vi "Transfer Packets From Host.vi"(1 "reset":bool, 2 "common resources":T13={"sync pulse resources"={"sync pulse destination terminal"="", "sync100"="", "sync pulse source terminal"="", "imported sync pulse register"="", "generate sync pulse handshake"="", "enable sync pulse register"="", "sync pulse clock"=""}, "serial channel resources"={"sc 0"={"completed frames register"=""}, "sc 1"={"completed frames register"=""}, "sc 2"={"completed frames register"=""}, "sc 3"={"completed frames register"=""}, "sc 4"={"completed frames register"=""}, "sc 5"={"completed frames register"=""}, "sc 6"={"completed frames register"=""}, "sc 7"={"completed frames register"=""}}, "dram manager 0"={"DRAM class"=refnum, "process clock"="", "registers"={"configuration"={"write time slice"="", "request time slice"="", "DRAM arbiter config"="", "partition config"=""}, "reset"={"handshake"={"start.go"="", "start.go rcvd"="", "done.go"="", "done.go rcvd"=""}, "process"={"in"="", "out"=""}, "write"={"in"="", "out 0"="", "out 1"="", "out 2"="", "out 3"=""}, "read"={"in"="", "out 0"="", "out 1"="", "out 2"="", "out 3"=""}}, "status"={"partition full"=""}}, "FIFOs"={"write data"={"FIFO 0"="", "FIFO 1"="", "FIFO 2"="", "FIFO 3"=""}, "request metadata"={"FIFO"=""}, "read data VOQ"={"FIFO 0"="", "FIFO 1"="", "FIFO 2"="", "FIFO 3"=""}, "read data"={"FIFO 0"="", "FIFO 1"="", "FIFO 2"="", "FIFO 3"=""}}, "num active streams"=0.0, "max open read requests"=256}, "dram manager 1"={"DRAM class"=refnum, "process clock"="", "registers"={"configuration"={"write time slice"="", "request time slice"="", "DRAM arbiter config"="", "partition config"=""}, "reset"={"handshake"={"start.go"="", "start.go rcvd"="", "done.go"="", "done.go rcvd"=""}, "process"={"in"="", "out"=""}, "write"={"in"="", "out 0"="", "out 1"="", "out 2"="", "out 3"=""}, "read"={"in"="", "out 0"="", "out 1"="", "out 2"="", "out 3"=""}}, "status"={"partition full"=""}}, "FIFOs"={"write data"={"FIFO 0"="", "FIFO 1"="", "FIFO 2"="", "FIFO 3"=""}, "request metadata"={"FIFO"=""}, "read data VOQ"={"FIFO 0"="", "FIFO 1"="", "FIFO 2"="", "FIFO 3"=""}, "read data"={"FIFO 0"="", "FIFO 1"="", "FIFO 2"="", "FIFO 3"=""}}, "num active streams"=0.0, "max open read requests"=256}}, 11 "dram partition configs":T12[](array[typedef])=[{"first address"=0, "last address"=0}, {"first address"=0, "last address"=0}, {"first address"=0, "last address"=0}, {"first address"=0, "last address"=0}, {"first address"=0, "last address"=0}, {"first address"=0, "last address"=0}, {"first address"=0, "last address"=0}, {"first address"=0, "last address"=0}], 12 "ready for output":bool[](array[boolean])=[TRUE, TRUE, TRUE, TRUE, TRUE, TRUE, TRUE, TRUE], 13 "channel configs":T24[](array[typedef])) -> (4 "tagged llp packets cluster":T1, 6 "end of data":bool[](array[boolean]), 8 "dram status":T11[](array[typedef]), 10 "output valid":bool[](array[boolean]))   [LabVIEW 2020, in "GettingStarted_Gen_148X_FPGA.lvlib"]
uses:
  GettingStarted_Gen_148X_FPGA.lvlib
  Types/Serial Output Channel Datapath Configuration.ctl
  Common/Types/Common Resources.ctl
  <instrlib>/_niInstr/Memory/v1/FPGA/DRAM/niInstr Memory DRAM v1 FPGA.lvclass
  <instrlib>/FlexRIO/CSI-2/v2/FPGA/Types/Sync Pulse Resources.ctl
  Common/Types/Serial Channel Resources.ctl
  Common/Types/Single Serial Channel Resources.ctl
  <instrlib>/FlexRIO/CSI-2/v2/FPGA/DRAM Manager/Private/DRAM Manager.ctl
  <instrlib>/FlexRIO/CSI-2/v2/FPGA/DRAM Manager/Private/Common/DRAM Manager Registers.ctl
  <instrlib>/FlexRIO/CSI-2/v2/FPGA/DRAM Manager/Private/Common/Handshake Registers.ctl
  <instrlib>/FlexRIO/CSI-2/v2/FPGA/DRAM Manager/Private/Common/DRAM Manager FIFOs.ctl
  <instrlib>/FlexRIO/CSI-2/v2/FPGA/DRAM Manager/Private/Common/Write Data FIFO Ref.ctl
  <instrlib>/FlexRIO/CSI-2/v2/FPGA/DRAM Manager/Private/Common/Read Request Metadata FIFO Ref.ctl
  <instrlib>/FlexRIO/CSI-2/v2/FPGA/DRAM Manager/Private/Common/Read Data FIFO Ref.ctl
  <instrlib>/FlexRIO/CSI-2/v2/FPGA/DRAM Manager/Public/Partition Range.ctl
  Common/Types/DRAM Status.ctl
  Common/Types/Tagged LLP Packets Cluster.ctl
  <instrlib>/FlexRIO/CSI-2/v2/FPGA/Types/Tagged LLP Packet.ctl
  <instrlib>/FlexRIO/CSI-2/v2/FPGA/Types/FPGA LLP Packet Tag.ctl
  <instrlib>/FlexRIO/CSI-2/v2/FPGA/Types/FPGA LLP Packet Timestamp.ctl
  <instrlib>/FlexRIO/CSI-2/v2/FPGA/Types/Timestamp ID.ctl
  <instrlib>/FlexRIO/CSI-2/v2/FPGA/Types/FPGA LLP Packet Size.ctl
  <instrlib>/FlexRIO/CSI-2/v2/FPGA/Types/LLP Packet.ctl
  <instrlib>/FlexRIO/CSI-2/v2/FPGA/Types/LLP Packet Header.ctl
  <instrlib>/FlexRIO/CSI-2/v2/FPGA/Types/LLP Packet Payload.ctl
  <instrlib>/FlexRIO/CSI-2/v2/FPGA/Types/LLP Packet Footer.ctl
  <instrlib>/_niInstr/Basic Elements/v1/FPGA/niInstr Basic Elements v1 FPGA.lvlib
  <instrlib>/FlexRIO/CSI-2/v2/FPGA/NI CSI-2 API FPGA v2.lvlib
  Common/GettingStarted_Common_148X_FPGA.lvlib
  <instrlib>/FlexRIO/CSI-2/v2/FPGA/DRAM Manager/DRAM Manager v2.lvlib
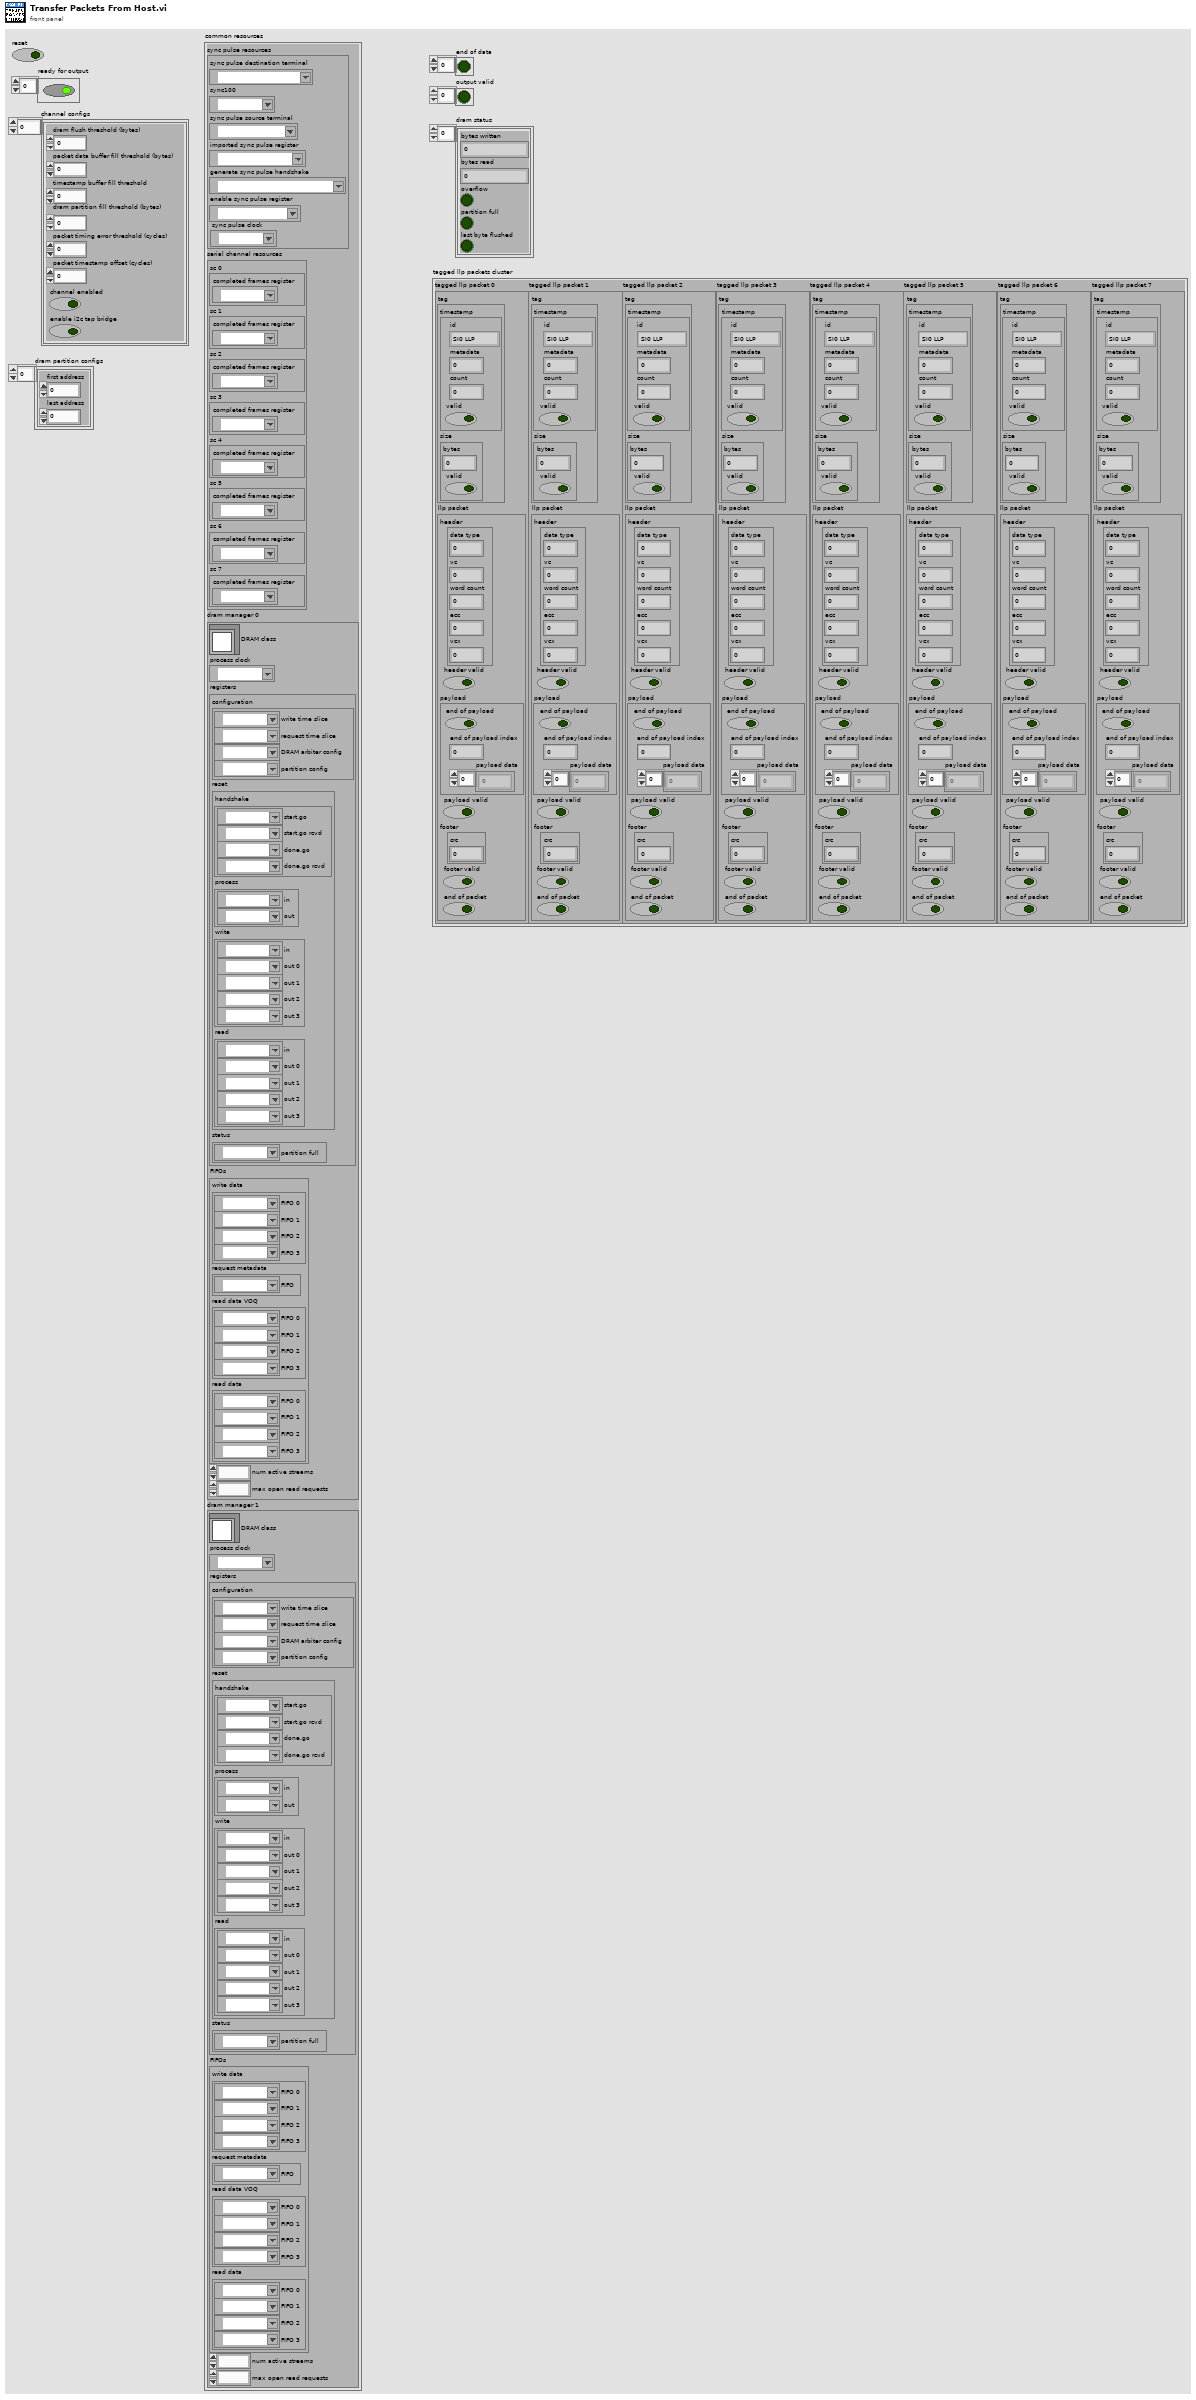
[diagram p1: front panel]
types:
  T1 = typedef "GettingStarted_Common_148X_FPGA.lvlib/Tagged LLP Packets Cluster.ctl" = cluster{"tagged llp packet 0":T2, "tagged llp packet 1":T2, "tagged llp packet 2":T2, "tagged llp packet 3":T2, "tagged llp packet 4":T2, "tagged llp packet 5":T2, "tagged llp packet 6":T2, "tagged llp packet 7":T2}
  T2 = typedef "NI CSI-2 API FPGA v2.lvlib/Tagged LLP Packet.ctl" = cluster{"tag":T3, "llp packet":T7}
  T3 = typedef "NI CSI-2 API FPGA v2.lvlib/FPGA LLP Packet Tag.ctl" = cluster{"timestamp":T4, "size":T6}
  T4 = typedef "NI CSI-2 API FPGA v2.lvlib/FPGA LLP Packet Timestamp.ctl" = cluster{"valid":bool, "count":fxp<+,50,50>, "id":T5, "metadata":u8}
  T5 = typedef "NI CSI-2 API FPGA v2.lvlib/Timestamp ID.ctl" = enum8{"SI0 LLP", "SI1 LLP", "SI2 LLP", "SI3 LLP", "SI4 LLP", "SI5 LLP", "SI6 LLP", "SI7 LLP", "SO0 LLP", "SO1 LLP", "SO2 LLP", "SO3 LLP", "SO4 LLP", "SO5 LLP", "SO6 LLP", "SO7 LLP", "Ser0 GPIO Bank", "Ser1 GPIO Bank", "Ser2 GPIO Bank", "Ser3 GPIO Bank", "Ser4 GPIO Bank", "Ser5 GPIO Bank", "Ser6 GPIO Bank", "Ser7 GPIO Bank", "Des0 GPIO Bank", "Des1 GPIO Bank", "Des2 GPIO Bank", "Des3 GPIO Bank", "Des4 GPIO Bank", "Des5 GPIO Bank", "Des6 GPIO Bank", "Des7 GPIO Bank", "User0", "User1", "User2", "User3", "User4", "User5", "User6", "User7", "User8", "User9", "User10", "User11", "User12", "User13", "User14", "User15", "User16", "User17", "User18", "User19", "User20", "User21", "User22", "User23", "User24", "User25", "User26", "User27", "User28", "User29", "User30", "User31"}
  T6 = typedef "NI CSI-2 API FPGA v2.lvlib/FPGA LLP Packet Size.ctl" = cluster{"bytes":fxp<+,17,17>, "valid":bool}
  T7 = typedef "NI CSI-2 API FPGA v2.lvlib/LLP Packet.ctl" = cluster{"header":T8, "header valid":bool, "payload":T9, "payload valid":bool, "footer":T10, "footer valid":bool, "end of packet":bool}
  T8 = typedef "NI CSI-2 API FPGA v2.lvlib/LLP Packet Header.ctl" = cluster{"word count":u16, "ecc":fxp<+,6,6>, "vcx":fxp<+,2,2>, "data type":fxp<+,6,6>, "vc":fxp<+,2,2>}
  T9 = typedef "NI CSI-2 API FPGA v2.lvlib/LLP Packet Payload.ctl" = cluster{"end of payload":bool, "end of payload index":fxp<+,3,3>, "payload data":u8[]}
  T10 = typedef "NI CSI-2 API FPGA v2.lvlib/LLP Packet Footer.ctl" = cluster{"crc":u16}
  T11 = typedef "GettingStarted_Common_148X_FPGA.lvlib/DRAM Status.ctl" = cluster{"bytes written":u64, "bytes read":u64, "overflow":bool, "partition full":bool, "last byte flushed":bool}
  T12 = typedef "DRAM Manager v2.lvlib/Partition Range.ctl" = cluster{"first address":u32, "last address":u32}
  T13 = typedef "GettingStarted_Common_148X_FPGA.lvlib/Common Resources.ctl" = cluster{"sync pulse resources":T14, "serial channel resources":T15, "dram manager 0":T17, "dram manager 1":T17}
  T14 = typedef "NI CSI-2 API FPGA v2.lvlib/Sync Pulse Resources.ctl" = cluster{"sync pulse destination terminal":refnum<k21>, "sync100":refnum<k21>, "sync pulse source terminal":refnum<k21>, "imported sync pulse register":refnum<k21>, "generate sync pulse handshake":refnum<k21>, "enable sync pulse register":refnum<k21>, "sync pulse clock":refnum<k21>}
  T15 = typedef "GettingStarted_Common_148X_FPGA.lvlib/Serial Channel Resources.ctl" = cluster{"sc 0":T16, "sc 1":T16, "sc 2":T16, "sc 3":T16, "sc 4":T16, "sc 5":T16, "sc 6":T16, "sc 7":T16}
  T16 = typedef "GettingStarted_Common_148X_FPGA.lvlib/Single Serial Channel Resources.ctl" = cluster{"completed frames register":refnum<k21>}
  T17 = typedef "DRAM Manager v2.lvlib/DRAM Manager.ctl" = cluster{"DRAM class":refnum<class "niInstr Memory DRAM v1 FPGA.lvclass">, "process clock":refnum<k21>, "registers":T18, "FIFOs":T20, "num active streams":fxp<+,3,3>, "max open read requests":u16}
  T18 = typedef "DRAM Manager v2.lvlib/DRAM Manager Registers.ctl" = cluster{"configuration":cluster{"write time slice":refnum<k21>, "request time slice":refnum<k21>, "DRAM arbiter config":refnum<k21>, "partition config":refnum<k21>}, "reset":cluster{"handshake":T19, "process":cluster{"in":refnum<k21>, "out":refnum<k21>}, "write":cluster{"in":refnum<k21>, "out 0":refnum<k21>, "out 1":refnum<k21>, "out 2":refnum<k21>, "out 3":refnum<k21>}, "read":cluster{"in":refnum<k21>, "out 0":refnum<k21>, "out 1":refnum<k21>, "out 2":refnum<k21>, "out 3":refnum<k21>}}, "status":cluster{"partition full":refnum<k21>}}
  T19 = typedef "DRAM Manager v2.lvlib/Handshake Registers.ctl" = cluster{"start.go":refnum<k21>, "start.go rcvd":refnum<k21>, "done.go":refnum<k21>, "done.go rcvd":refnum<k21>}
  T20 = typedef "DRAM Manager v2.lvlib/DRAM Manager FIFOs.ctl" = cluster{"write data":cluster{"FIFO 0":T21, "FIFO 1":T21, "FIFO 2":T21, "FIFO 3":T21}, "request metadata":cluster{"FIFO":T22}, "read data VOQ":cluster{"FIFO 0":T23, "FIFO 1":T23, "FIFO 2":T23, "FIFO 3":T23}, "read data":cluster{"FIFO 0":T23, "FIFO 1":T23, "FIFO 2":T23, "FIFO 3":T23}}
  T21 = typedef "DRAM Manager v2.lvlib/Write Data FIFO Ref.ctl" = refnum<k21>
  T22 = typedef "DRAM Manager v2.lvlib/Read Request Metadata FIFO Ref.ctl" = refnum<k21>
  T23 = typedef "DRAM Manager v2.lvlib/Read Data FIFO Ref.ctl" = refnum<k21>
  T24 = typedef "GettingStarted_Gen_148X_FPGA.lvlib/Serial Output Channel Datapath Configuration.ctl" = cluster{"dram flush threshold (bytes)":u64, "packet data buffer fill threshold (bytes)":u64, "timestamp buffer fill threshold":u32, "packet timing error threshold (cycles)":u64, "channel enabled":bool, "dram partition fill threshold (bytes)":u64, "enable i2c tap bridge":bool, "packet timestamp offset (cycles)":i64}
  T25 = typedef "GettingStarted_Gen_148X_FPGA.lvlib/8 Out DRAM Resources.ctl" = cluster{"so 0 resources":T26, "so 1 resources":T26, "so 2 resources":T26, "so 3 resources":T26, "so 4 resources":T26, "so 5 resources":T26, "so 6 resources":T26, "so 7 resources":T26}
  T26 = typedef "GettingStarted_Gen_148X_FPGA.lvlib/Serial Output DRAM Resources.ctl" = cluster{"dram manager":T17, "llp packets dma fifo":refnum<k21>, "dram stream id":fxp<+,2,2>}
  T27 = cluster{"end of data":bool, "dram status":T11, "output valid":bool}
  T28 = cluster{"end of data":bool, "dram status":T11, "output valid":bool}[]
  T29 = typedef "GettingStarted_Gen_148X_FPGA.lvlib/4 In 4 Out DRAM Resources.ctl" = cluster{"so 0 resources":T26, "so 1 resources":T26, "so 2 resources":T26, "so 3 resources":T26}
  T30 = typedef "GettingStarted_Gen_148X_FPGA.lvlib/2 In 2 Out DRAM Resources.ctl" = cluster{"so 0 resources":T26, "so 1 resources":T26}
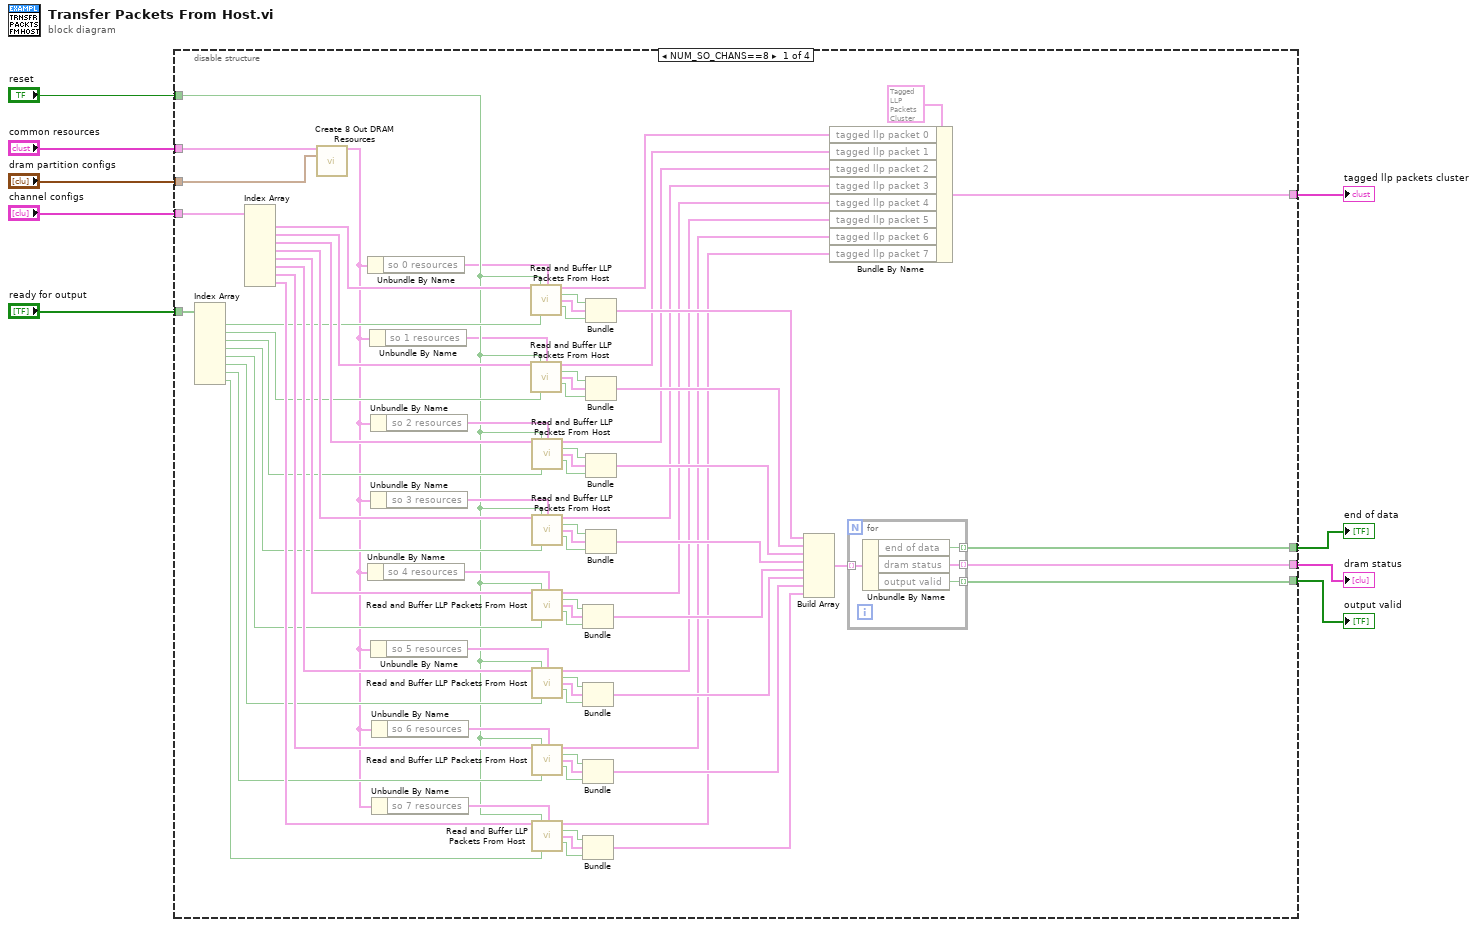
[diagram p0: block diagram]
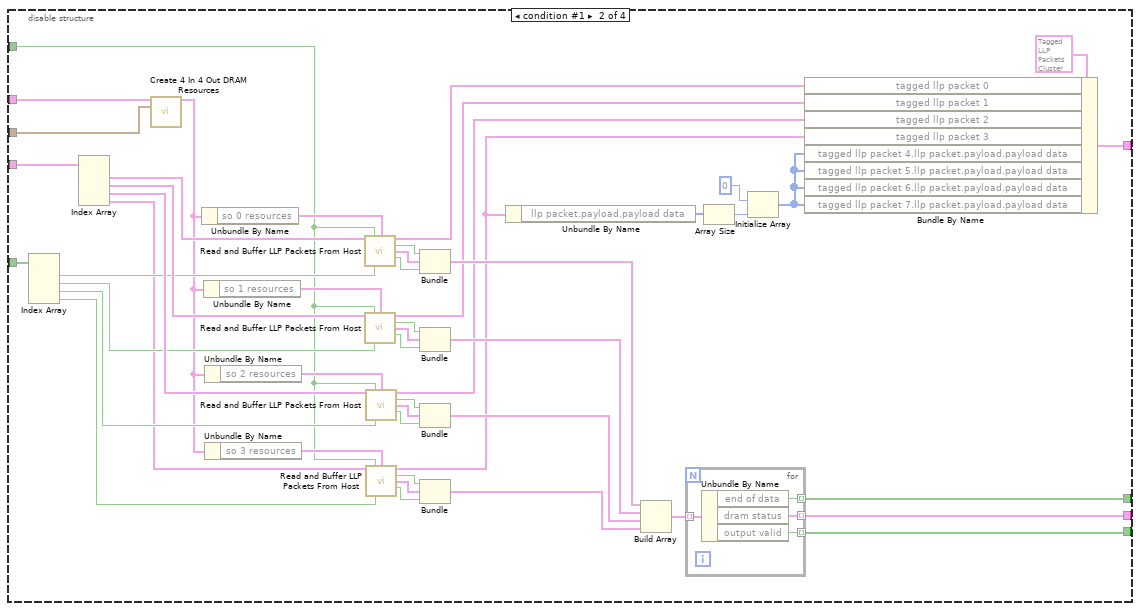
[diagram p2: hidden frame]
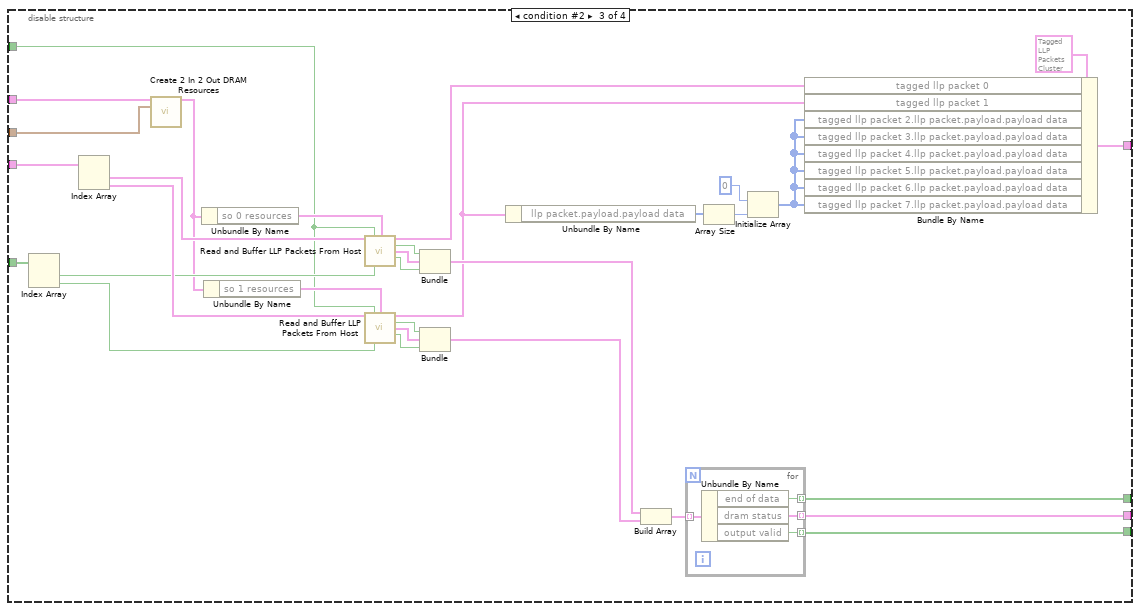
[diagram p3: hidden frame]
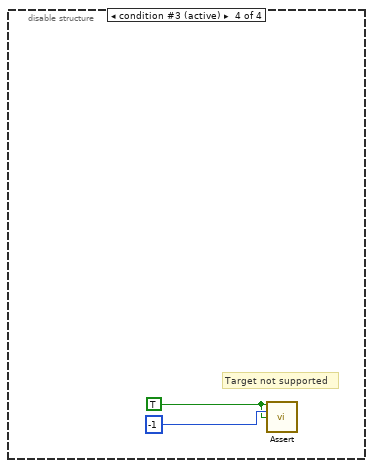
[diagram p4: hidden frame]
diagram:
  n1 = disable-structure shown="NUM_SO_CHANS==8" {
    disable-tunnel: "channel configs" -> [w85 w137 w173 _]
    disable-tunnel: "common resources" -> [w60 w125 w164 _]
    disable-tunnel: "dram partition configs" -> [w61 w126 w165 _]
    disable-tunnel: "ready for output" -> [w84 w136 w172 _]
    disable-tunnel: [w25 w110 w153 _] -> w6
    disable-tunnel: "reset" -> [w24 w102 w152 _]
    disable-tunnel: [w21 w100 w150 _] -> w3
    disable-tunnel: [w20 w101 w151 _] -> w2
    disable-tunnel: [w10 w98 w148 _] -> w1
    frame condition #0 {
      n2 = Index Array(array=w84) -> (element #1=w69:bool, element #2=w68:bool, element #3=w62:bool, element #4=w63:bool, element #5=w64:bool, element #6=w65:bool, element #7=w66:bool, element #8=w67:bool)  [unwired: 8 in]
      n3 = Index Array(array=w85) -> (element #1=w83:T24, element #2=w82:T24, element #3=w80:T24, element #4=w81:T24, element #5=w70:T24, element #6=w71:T24, element #7=w72:T24, element #8=w73:T24)  [unwired: 8 in]
      n4 = call "Create 8 Out DRAM Resources.vi"("common resources"=w60, "dram partition configs"=w61) -> ("channel dram resources"=w59:T25)  [unwired: 13 in]
      n5 = Unbundle By Name(w59) -> ("so 0 resources"=w23:T26)
      n6 = Unbundle By Name(w59) -> ("so 4 resources"=w77:T26)
      n7 = Unbundle By Name(w59) -> ("so 1 resources"=w22:T26)
      n8 = Unbundle By Name(w59) -> ("so 2 resources"=w79:T26)
      n9 = Unbundle By Name(w59) -> ("so 3 resources"=w78:T26)
      n10 = Unbundle By Name(w59) -> ("so 5 resources"=w76:T26)
      n11 = Unbundle By Name(w59) -> ("so 6 resources"=w75:T26)
      n12 = Unbundle By Name(w59) -> ("so 7 resources"=w74:T26)
      n13 = call "Read and Buffer LLP Packets From Host.vi"("channel configuration"=w83, "reset"=w24, "resources"=w23, "ready for output"=w69) -> ("tagged llp packet"=w11:T2, "end of data"=w58:bool, "dram status"=w57:T11, "output valid"=w56:bool)  [unwired: 8 in]
      n14 = call "Read and Buffer LLP Packets From Host.vi"("channel configuration"=w82, "reset"=w24, "resources"=w22, "ready for output"=w68) -> ("tagged llp packet"=w12:T2, "end of data"=w53:bool, "dram status"=w54:T11, "output valid"=w55:bool)  [unwired: 8 in]
      n15 = call "Read and Buffer LLP Packets From Host.vi"("channel configuration"=w80, "reset"=w24, "resources"=w79, "ready for output"=w62) -> ("tagged llp packet"=w13:T2, "end of data"=w52:bool, "dram status"=w51:T11, "output valid"=w50:bool)  [unwired: 8 in]
      n16 = call "Read and Buffer LLP Packets From Host.vi"("channel configuration"=w81, "reset"=w24, "resources"=w78, "ready for output"=w63) -> ("tagged llp packet"=w14:T2, "end of data"=w49:bool, "dram status"=w48:T11, "output valid"=w47:bool)  [unwired: 8 in]
      n17 = call "Read and Buffer LLP Packets From Host.vi"("channel configuration"=w70, "reset"=w24, "resources"=w77, "ready for output"=w64) -> ("tagged llp packet"=w15:T2, "end of data"=w46:bool, "dram status"=w45:T11, "output valid"=w44:bool)  [unwired: 8 in]
      n18 = call "Read and Buffer LLP Packets From Host.vi"("channel configuration"=w71, "reset"=w24, "resources"=w76, "ready for output"=w65) -> ("tagged llp packet"=w16:T2, "end of data"=w43:bool, "dram status"=w42:T11, "output valid"=w41:bool)  [unwired: 8 in]
      n19 = call "Read and Buffer LLP Packets From Host.vi"("channel configuration"=w72, "reset"=w24, "resources"=w75, "ready for output"=w66) -> ("tagged llp packet"=w17:T2, "end of data"=w40:bool, "dram status"=w39:T11, "output valid"=w38:bool)  [unwired: 8 in]
      n20 = call "Read and Buffer LLP Packets From Host.vi"("channel configuration"=w73, "reset"=w24, "resources"=w74, "ready for output"=w67) -> ("tagged llp packet"=w18:T2, "end of data"=w37:bool, "dram status"=w36:T11, "output valid"=w35:bool)  [unwired: 8 in]
      n21 = Bundle("end of data"=w46, "dram status"=w45, "output valid"=w44) -> (w30:T27)  [unwired: 1 in]
      n22 = Bundle("end of data"=w43, "dram status"=w42, "output valid"=w41) -> (w29:T27)  [unwired: 1 in]
      n23 = Bundle("end of data"=w40, "dram status"=w39, "output valid"=w38) -> (w28:T27)  [unwired: 1 in]
      n24 = Bundle("end of data"=w37, "dram status"=w36, "output valid"=w35) -> (w27:T27)  [unwired: 1 in]
      n25 = Bundle("end of data"=w58, "dram status"=w57, "output valid"=w56) -> (w34:T27)  [unwired: 1 in]
      n26 = Bundle("end of data"=w53, "dram status"=w54, "output valid"=w55) -> (w33:T27)  [unwired: 1 in]
      n27 = Bundle("end of data"=w52, "dram status"=w51, "output valid"=w50) -> (w32:T27)  [unwired: 1 in]
      n28 = Bundle("end of data"=w49, "dram status"=w48, "output valid"=w47) -> (w31:T27)  [unwired: 1 in]
      n29 = Build Array(w34, w33, w32, w31, w30, w29, w28, w27) -> (w26:T28)
      n30 = Bundle By Name(cluster=T1 {"tagged llp packet 0"={"tag"={"timestamp"={"valid"=FALSE, "count"=0.0, "id"=enum."SI0 LLP", "metadata"=0}, "size"={"bytes"=0.0, "valid"=FALSE}}, "llp packet"={"header"={"word count"=0, "ecc"=0.0, "vcx"=0.0, "data type"=0.0, "vc"=0.0}, "header valid"=FALSE, "payload"={"end of payload"=FALSE, "end of payload index"=0.0, "payload data"=[0, 0, 0, 0]}, "payload valid"=FALSE, "footer"={"crc"=0}, "footer valid"=FALSE, "end of packet"=FALSE}}, "tagged llp packet 1"={"tag"={"timestamp"={"valid"=FALSE, "count"=0.0, "id"=enum."SI0 LLP", "metadata"=0}, "size"={"bytes"=0.0, "valid"=FALSE}}, "llp packet"={"header"={"word count"=0, "ecc"=0.0, "vcx"=0.0, "data type"=0.0, "vc"=0.0}, "header valid"=FALSE, "payload"={"end of payload"=FALSE, "end of payload index"=0.0, "payload data"=[0, 0, 0, 0]}, "payload valid"=FALSE, "footer"={"crc"=0}, "footer valid"=FALSE, "end of packet"=FALSE}}, "tagged llp packet 2"={"tag"={"timestamp"={"valid"=FALSE, "count"=0.0, "id"=enum."SI0 LLP", "metadata"=0}, "size"={"bytes"=0.0, "valid"=FALSE}}, "llp packet"={"header"={"word count"=0, "ecc"=0.0, "vcx"=0.0, "data type"=0.0, "vc"=0.0}, "header valid"=FALSE, "payload"={"end of payload"=FALSE, "end of payload index"=0.0, "payload data"=[0, 0, 0, 0]}, "payload valid"=FALSE, "footer"={"crc"=0}, "footer valid"=FALSE, "end of packet"=FALSE}}, "tagged llp packet 3"={"tag"={"timestamp"={"valid"=FALSE, "count"=0.0, "id"=enum."SI0 LLP", "metadata"=0}, "size"={"bytes"=0.0, "valid"=FALSE}}, "llp packet"={"header"={"word count"=0, "ecc"=0.0, "vcx"=0.0, "data type"=0.0, "vc"=0.0}, "header valid"=FALSE, "payload"={"end of payload"=FALSE, "end of payload index"=0.0, "payload data"=[0, 0, 0, 0]}, "payload valid"=FALSE, "footer"={"crc"=0}, "footer valid"=FALSE, "end of packet"=FALSE}}, "tagged llp packet 4"={"tag"={"timestamp"={"valid"=FALSE, "count"=0.0, "id"=enum."SI0 LLP", "metadata"=0}, "size"={"bytes"=0.0, "valid"=FALSE}}, "llp packet"={"header"={"word count"=0, "ecc"=0.0, "vcx"=0.0, "data type"=0.0, "vc"=0.0}, "header valid"=FALSE, "payload"={"end of payload"=FALSE, "end of payload index"=0.0, "payload data"=[0, 0, 0, 0]}, "payload valid"=FALSE, "footer"={"crc"=0}, "footer valid"=FALSE, "end of packet"=FALSE}}, "tagged llp packet 5"={"tag"={"timestamp"={"valid"=FALSE, "count"=0.0, "id"=enum."SI0 LLP", "metadata"=0}, "size"={"bytes"=0.0, "valid"=FALSE}}, "llp packet"={"header"={"word count"=0, "ecc"=0.0, "vcx"=0.0, "data type"=0.0, "vc"=0.0}, "header valid"=FALSE, "payload"={"end of payload"=FALSE, "end of payload index"=0.0, "payload data"=[0, 0, 0, 0]}, "payload valid"=FALSE, "footer"={"crc"=0}, "footer valid"=FALSE, "end of packet"=FALSE}}, "tagged llp packet 6"={"tag"={"timestamp"={"valid"=FALSE, "count"=0.0, "id"=enum."SI0 LLP", "metadata"=0}, "size"={"bytes"=0.0, "valid"=FALSE}}, "llp packet"={"header"={"word count"=0, "ecc"=0.0, "vcx"=0.0, "data type"=0.0, "vc"=0.0}, "header valid"=FALSE, "payload"={"end of payload"=FALSE, "end of payload index"=0.0, "payload data"=[0, 0, 0, 0]}, "payload valid"=FALSE, "footer"={"crc"=0}, "footer valid"=FALSE, "end of packet"=FALSE}}, "tagged llp packet 7"={"tag"={"timestamp"={"valid"=FALSE, "count"=0.0, "id"=enum."SI0 LLP", "metadata"=0}, "size"={"bytes"=0.0, "valid"=FALSE}}, "llp packet"={"header"={"word count"=0, "ecc"=0.0, "vcx"=0.0, "data type"=0.0, "vc"=0.0}, "header valid"=FALSE, "payload"={"end of payload"=FALSE, "end of payload index"=0.0, "payload data"=[0, 0, 0, 0]}, "payload valid"=FALSE, "footer"={"crc"=0}, "footer valid"=FALSE, "end of packet"=FALSE}}} ("tagged llp packets cluster"), "tagged llp packet 0"=w11, "tagged llp packet 1"=w12, "tagged llp packet 2"=w13, "tagged llp packet 3"=w14, "tagged llp packet 4"=w15, "tagged llp packet 5"=w16, "tagged llp packet 6"=w17, "tagged llp packet 7"=w18) -> (w10:T1)
      n31 = for {
        tunnel: w26 -> [w89] mode=indexing
        tunnel: [w88] -> w20 mode=indexing
        tunnel: [w87] -> w25 mode=indexing
        tunnel: [w86] -> w21 mode=indexing
        n32 = Unbundle By Name(w89) -> ("end of data"=w88:bool, "dram status"=w87:T11, "output valid"=w86:bool)
      }
    }
    frame condition #1 {
      n33 = Index Array(array=w136) -> (element #1=w129:bool, element #2=w128:bool, element #3=w127:bool, element #4=w103:bool)  [unwired: 4 in]
      n34 = Index Array(array=w137) -> (element #1=w134:T24, element #2=w132:T24, element #3=w131:T24, element #4=w106:T24)  [unwired: 4 in]
      n35 = call "Create 4 In 4 Out DRAM Resources.vi"("common resources"=w125, "dram partition configs"=w126) -> ("channel dram resources"=w124:T29)  [unwired: 13 in]
      n36 = Unbundle By Name(w124) -> ("so 0 resources"=w135:T26)
      n37 = Unbundle By Name(w124) -> ("so 1 resources"=w133:T26)
      n38 = Unbundle By Name(w124) -> ("so 2 resources"=w130:T26)
      n39 = Unbundle By Name(w124) -> ("so 3 resources"=w104:T26)
      n40 = call "Read and Buffer LLP Packets From Host.vi"("channel configuration"=w134, "reset"=w102, "resources"=w135, "ready for output"=w129) -> ("tagged llp packet"=w95:T2, "end of data"=w123:bool, "dram status"=w122:T11, "output valid"=w121:bool)  [unwired: 8 in]
      n41 = call "Read and Buffer LLP Packets From Host.vi"("channel configuration"=w132, "reset"=w102, "resources"=w133, "ready for output"=w128) -> ("tagged llp packet"=w96:T2, "end of data"=w118:bool, "dram status"=w119:T11, "output valid"=w120:bool)  [unwired: 8 in]
      n42 = call "Read and Buffer LLP Packets From Host.vi"("channel configuration"=w131, "reset"=w102, "resources"=w130, "ready for output"=w127) -> ("tagged llp packet"=w97:T2, "end of data"=w117:bool, "dram status"=w116:T11, "output valid"=w115:bool)  [unwired: 8 in]
      n43 = call "Read and Buffer LLP Packets From Host.vi"("channel configuration"=w106, "reset"=w102, "resources"=w104, "ready for output"=w103) -> ("tagged llp packet"=w90:T2, "end of data"=w109:bool, "dram status"=w108:T11, "output valid"=w107:bool)  [unwired: 8 in]
      n44 = Bundle("end of data"=w123, "dram status"=w122, "output valid"=w121) -> (w114:T27)  [unwired: 1 in]
      n45 = Bundle("end of data"=w118, "dram status"=w119, "output valid"=w120) -> (w113:T27)  [unwired: 1 in]
      n46 = Bundle("end of data"=w117, "dram status"=w116, "output valid"=w115) -> (w112:T27)  [unwired: 1 in]
      n47 = Bundle("end of data"=w109, "dram status"=w108, "output valid"=w107) -> (w105:T27)  [unwired: 1 in]
      n48 = Unbundle By Name(w90) -> ("llp packet.payload.payload data"=w94:u8[])
      n49 = Build Array(w114, w113, w112, w105) -> (w111:T28)
      n50 = for {
        tunnel: w111 -> [w141] mode=indexing
        tunnel: [w140] -> w101 mode=indexing
        tunnel: [w139] -> w110 mode=indexing
        tunnel: [w138] -> w100 mode=indexing
        n51 = Unbundle By Name(w141) -> ("end of data"=w140:bool, "dram status"=w139:T11, "output valid"=w138:bool)
      }
      n52 = Array Size(array=w94) -> (size(s)=w93:i32)
      n53 = Initialize Array(u8 0 ("element"), w93) -> (w91:u8[])
      n54 = Bundle By Name(cluster=T1 {"tagged llp packet 0"={"tag"={"timestamp"={"valid"=FALSE, "count"=0.0, "id"=enum."SI0 LLP", "metadata"=0}, "size"={"bytes"=0.0, "valid"=FALSE}}, "llp packet"={"header"={"word count"=0, "ecc"=0.0, "vcx"=0.0, "data type"=0.0, "vc"=0.0}, "header valid"=FALSE, "payload"={"end of payload"=FALSE, "end of payload index"=0.0, "payload data"=[0, 0, 0, 0]}, "payload valid"=FALSE, "footer"={"crc"=0}, "footer valid"=FALSE, "end of packet"=FALSE}}, "tagged llp packet 1"={"tag"={"timestamp"={"valid"=FALSE, "count"=0.0, "id"=enum."SI0 LLP", "metadata"=0}, "size"={"bytes"=0.0, "valid"=FALSE}}, "llp packet"={"header"={"word count"=0, "ecc"=0.0, "vcx"=0.0, "data type"=0.0, "vc"=0.0}, "header valid"=FALSE, "payload"={"end of payload"=FALSE, "end of payload index"=0.0, "payload data"=[0, 0, 0, 0]}, "payload valid"=FALSE, "footer"={"crc"=0}, "footer valid"=FALSE, "end of packet"=FALSE}}, "tagged llp packet 2"={"tag"={"timestamp"={"valid"=FALSE, "count"=0.0, "id"=enum."SI0 LLP", "metadata"=0}, "size"={"bytes"=0.0, "valid"=FALSE}}, "llp packet"={"header"={"word count"=0, "ecc"=0.0, "vcx"=0.0, "data type"=0.0, "vc"=0.0}, "header valid"=FALSE, "payload"={"end of payload"=FALSE, "end of payload index"=0.0, "payload data"=[0, 0, 0, 0]}, "payload valid"=FALSE, "footer"={"crc"=0}, "footer valid"=FALSE, "end of packet"=FALSE}}, "tagged llp packet 3"={"tag"={"timestamp"={"valid"=FALSE, "count"=0.0, "id"=enum."SI0 LLP", "metadata"=0}, "size"={"bytes"=0.0, "valid"=FALSE}}, "llp packet"={"header"={"word count"=0, "ecc"=0.0, "vcx"=0.0, "data type"=0.0, "vc"=0.0}, "header valid"=FALSE, "payload"={"end of payload"=FALSE, "end of payload index"=0.0, "payload data"=[0, 0, 0, 0]}, "payload valid"=FALSE, "footer"={"crc"=0}, "footer valid"=FALSE, "end of packet"=FALSE}}, "tagged llp packet 4"={"tag"={"timestamp"={"valid"=FALSE, "count"=0.0, "id"=enum."SI0 LLP", "metadata"=0}, "size"={"bytes"=0.0, "valid"=FALSE}}, "llp packet"={"header"={"word count"=0, "ecc"=0.0, "vcx"=0.0, "data type"=0.0, "vc"=0.0}, "header valid"=FALSE, "payload"={"end of payload"=FALSE, "end of payload index"=0.0, "payload data"=[0, 0, 0, 0]}, "payload valid"=FALSE, "footer"={"crc"=0}, "footer valid"=FALSE, "end of packet"=FALSE}}, "tagged llp packet 5"={"tag"={"timestamp"={"valid"=FALSE, "count"=0.0, "id"=enum."SI0 LLP", "metadata"=0}, "size"={"bytes"=0.0, "valid"=FALSE}}, "llp packet"={"header"={"word count"=0, "ecc"=0.0, "vcx"=0.0, "data type"=0.0, "vc"=0.0}, "header valid"=FALSE, "payload"={"end of payload"=FALSE, "end of payload index"=0.0, "payload data"=[0, 0, 0, 0]}, "payload valid"=FALSE, "footer"={"crc"=0}, "footer valid"=FALSE, "end of packet"=FALSE}}, "tagged llp packet 6"={"tag"={"timestamp"={"valid"=FALSE, "count"=0.0, "id"=enum."SI0 LLP", "metadata"=0}, "size"={"bytes"=0.0, "valid"=FALSE}}, "llp packet"={"header"={"word count"=0, "ecc"=0.0, "vcx"=0.0, "data type"=0.0, "vc"=0.0}, "header valid"=FALSE, "payload"={"end of payload"=FALSE, "end of payload index"=0.0, "payload data"=[0, 0, 0, 0]}, "payload valid"=FALSE, "footer"={"crc"=0}, "footer valid"=FALSE, "end of packet"=FALSE}}, "tagged llp packet 7"={"tag"={"timestamp"={"valid"=FALSE, "count"=0.0, "id"=enum."SI0 LLP", "metadata"=0}, "size"={"bytes"=0.0, "valid"=FALSE}}, "llp packet"={"header"={"word count"=0, "ecc"=0.0, "vcx"=0.0, "data type"=0.0, "vc"=0.0}, "header valid"=FALSE, "payload"={"end of payload"=FALSE, "end of payload index"=0.0, "payload data"=[0, 0, 0, 0]}, "payload valid"=FALSE, "footer"={"crc"=0}, "footer valid"=FALSE, "end of packet"=FALSE}}} ("tagged llp packets cluster"), "tagged llp packet 0"=w95, "tagged llp packet 1"=w96, "tagged llp packet 2"=w97, "tagged llp packet 3"=w90, "tagged llp packet 4.llp packet.payload.payload data"=w91, "tagged llp packet 5.llp packet.payload.payload data"=w91, "tagged llp packet 6.llp packet.payload.payload data"=w91, "tagged llp packet 7.llp packet.payload.payload data"=w91) -> (w98:T1)
    }
    frame condition #2 {
      n55 = Index Array(array=w172) -> (element #1=w167:bool, element #2=w166:bool)  [unwired: 2 in]
      n56 = Index Array(array=w173) -> (element #1=w170:T24, element #2=w168:T24)  [unwired: 2 in]
      n57 = call "Create 2 In 2 Out DRAM Resources.vi"("common resources"=w164, "dram partition configs"=w165) -> ("channel dram resources"=w163:T30)  [unwired: 13 in]
      n58 = Unbundle By Name(w163) -> ("so 0 resources"=w171:T26)
      n59 = Unbundle By Name(w163) -> ("so 1 resources"=w169:T26)
      n60 = call "Read and Buffer LLP Packets From Host.vi"("channel configuration"=w170, "reset"=w152, "resources"=w171, "ready for output"=w167) -> ("tagged llp packet"=w147:T2, "end of data"=w162:bool, "dram status"=w161:T11, "output valid"=w160:bool)  [unwired: 8 in]
      n61 = call "Read and Buffer LLP Packets From Host.vi"("channel configuration"=w168, "reset"=w152, "resources"=w169, "ready for output"=w166) -> ("tagged llp packet"=w142:T2, "end of data"=w157:bool, "dram status"=w158:T11, "output valid"=w159:bool)  [unwired: 8 in]
      n62 = Bundle("end of data"=w162, "dram status"=w161, "output valid"=w160) -> (w156:T27)  [unwired: 1 in]
      n63 = Bundle("end of data"=w157, "dram status"=w158, "output valid"=w159) -> (w155:T27)  [unwired: 1 in]
      n64 = Unbundle By Name(w142) -> ("llp packet.payload.payload data"=w146:u8[])
      n65 = Build Array(w156, w155) -> (w154:T28)
      n66 = for {
        tunnel: w154 -> [w177] mode=indexing
        tunnel: [w176] -> w151 mode=indexing
        tunnel: [w175] -> w153 mode=indexing
        tunnel: [w174] -> w150 mode=indexing
        n67 = Unbundle By Name(w177) -> ("end of data"=w176:bool, "dram status"=w175:T11, "output valid"=w174:bool)
      }
      n68 = Array Size(array=w146) -> (size(s)=w145:i32)
      n69 = Initialize Array(u8 0 ("element"), w145) -> (w143:u8[])
      n70 = Bundle By Name(cluster=T1 {"tagged llp packet 0"={"tag"={"timestamp"={"valid"=FALSE, "count"=0.0, "id"=enum."SI0 LLP", "metadata"=0}, "size"={"bytes"=0.0, "valid"=FALSE}}, "llp packet"={"header"={"word count"=0, "ecc"=0.0, "vcx"=0.0, "data type"=0.0, "vc"=0.0}, "header valid"=FALSE, "payload"={"end of payload"=FALSE, "end of payload index"=0.0, "payload data"=[0, 0, 0, 0]}, "payload valid"=FALSE, "footer"={"crc"=0}, "footer valid"=FALSE, "end of packet"=FALSE}}, "tagged llp packet 1"={"tag"={"timestamp"={"valid"=FALSE, "count"=0.0, "id"=enum."SI0 LLP", "metadata"=0}, "size"={"bytes"=0.0, "valid"=FALSE}}, "llp packet"={"header"={"word count"=0, "ecc"=0.0, "vcx"=0.0, "data type"=0.0, "vc"=0.0}, "header valid"=FALSE, "payload"={"end of payload"=FALSE, "end of payload index"=0.0, "payload data"=[0, 0, 0, 0]}, "payload valid"=FALSE, "footer"={"crc"=0}, "footer valid"=FALSE, "end of packet"=FALSE}}, "tagged llp packet 2"={"tag"={"timestamp"={"valid"=FALSE, "count"=0.0, "id"=enum."SI0 LLP", "metadata"=0}, "size"={"bytes"=0.0, "valid"=FALSE}}, "llp packet"={"header"={"word count"=0, "ecc"=0.0, "vcx"=0.0, "data type"=0.0, "vc"=0.0}, "header valid"=FALSE, "payload"={"end of payload"=FALSE, "end of payload index"=0.0, "payload data"=[0, 0, 0, 0]}, "payload valid"=FALSE, "footer"={"crc"=0}, "footer valid"=FALSE, "end of packet"=FALSE}}, "tagged llp packet 3"={"tag"={"timestamp"={"valid"=FALSE, "count"=0.0, "id"=enum."SI0 LLP", "metadata"=0}, "size"={"bytes"=0.0, "valid"=FALSE}}, "llp packet"={"header"={"word count"=0, "ecc"=0.0, "vcx"=0.0, "data type"=0.0, "vc"=0.0}, "header valid"=FALSE, "payload"={"end of payload"=FALSE, "end of payload index"=0.0, "payload data"=[0, 0, 0, 0]}, "payload valid"=FALSE, "footer"={"crc"=0}, "footer valid"=FALSE, "end of packet"=FALSE}}, "tagged llp packet 4"={"tag"={"timestamp"={"valid"=FALSE, "count"=0.0, "id"=enum."SI0 LLP", "metadata"=0}, "size"={"bytes"=0.0, "valid"=FALSE}}, "llp packet"={"header"={"word count"=0, "ecc"=0.0, "vcx"=0.0, "data type"=0.0, "vc"=0.0}, "header valid"=FALSE, "payload"={"end of payload"=FALSE, "end of payload index"=0.0, "payload data"=[0, 0, 0, 0]}, "payload valid"=FALSE, "footer"={"crc"=0}, "footer valid"=FALSE, "end of packet"=FALSE}}, "tagged llp packet 5"={"tag"={"timestamp"={"valid"=FALSE, "count"=0.0, "id"=enum."SI0 LLP", "metadata"=0}, "size"={"bytes"=0.0, "valid"=FALSE}}, "llp packet"={"header"={"word count"=0, "ecc"=0.0, "vcx"=0.0, "data type"=0.0, "vc"=0.0}, "header valid"=FALSE, "payload"={"end of payload"=FALSE, "end of payload index"=0.0, "payload data"=[0, 0, 0, 0]}, "payload valid"=FALSE, "footer"={"crc"=0}, "footer valid"=FALSE, "end of packet"=FALSE}}, "tagged llp packet 6"={"tag"={"timestamp"={"valid"=FALSE, "count"=0.0, "id"=enum."SI0 LLP", "metadata"=0}, "size"={"bytes"=0.0, "valid"=FALSE}}, "llp packet"={"header"={"word count"=0, "ecc"=0.0, "vcx"=0.0, "data type"=0.0, "vc"=0.0}, "header valid"=FALSE, "payload"={"end of payload"=FALSE, "end of payload index"=0.0, "payload data"=[0, 0, 0, 0]}, "payload valid"=FALSE, "footer"={"crc"=0}, "footer valid"=FALSE, "end of packet"=FALSE}}, "tagged llp packet 7"={"tag"={"timestamp"={"valid"=FALSE, "count"=0.0, "id"=enum."SI0 LLP", "metadata"=0}, "size"={"bytes"=0.0, "valid"=FALSE}}, "llp packet"={"header"={"word count"=0, "ecc"=0.0, "vcx"=0.0, "data type"=0.0, "vc"=0.0}, "header valid"=FALSE, "payload"={"end of payload"=FALSE, "end of payload index"=0.0, "payload data"=[0, 0, 0, 0]}, "payload valid"=FALSE, "footer"={"crc"=0}, "footer valid"=FALSE, "end of packet"=FALSE}}} ("tagged llp packets cluster"), "tagged llp packet 0"=w147, "tagged llp packet 1"=w142, "tagged llp packet 2.llp packet.payload.payload data"=w143, "tagged llp packet 3.llp packet.payload.payload data"=w143, "tagged llp packet 4.llp packet.payload.payload data"=w143, "tagged llp packet 5.llp packet.payload.payload data"=w143, "tagged llp packet 6.llp packet.payload.payload data"=w143, "tagged llp packet 7.llp packet.payload.payload data"=w143) -> (w148:T1)
    }
    frame condition #3 (active) {
      w178 = TRUE ("assert")
      # "Target not supported"
      n71 = call <instrlib>:"Assert.vi"("assert"=w178, "error code"=-1, "enable show error"=w178) -> ()  [unwired: 13 in]
    }
  }
  "output valid" <- w3
  "dram status" <- w6
  "end of data" <- w2
  "tagged llp packets cluster" <- w1
